vi "Begin.vi"(8 "error in":errorcluster) -> (0 "error out":errorcluster)   [LabVIEW 2016]
doc: "Called before other user functions, this VI is expected to open initial I/O refnums, load in file data, and do all program initialization. Notice that the <B>error out</B> terminal is simply used for data flow. Wiring it to other structures or subVIs ensures that this VI runs first."
uses:
  <vilib>/Rock Robotics/WPI/SafetyOutput/WPI_SafetyOutputConfigMenu.ctl
  <vilib>/Rock Robotics/WPI/DriverStation/WPI_DriverStationRobotMode2.ctl
  <vilib>/Rock Robotics/WPI/Joystick/WPI_JoystickDeviceEnum.ctl
  <vilib>/Rock Robotics/SystemInterfaces/DIO/FPGA_DIOPWMChannel.ctl
  <vilib>/Rock Robotics/SystemInterfaces/DIO/FPGA_DIOChannel.ctl
  <vilib>/Rock Robotics/SystemInterfaces/i2clib/i2c_bus.ctl
  <vilib>/Rock Robotics/SystemInterfaces/DIO/FPGA_DIORelayChannel.ctl
  <vilib>/Rock Robotics/WPI/Relay/WPI_RelayDirection.ctl
  <vilib>/Rock Robotics/WPI/Solenoid/WPI_SolenoidChannel.ctl
  <vilib>/Rock Robotics/WPI/ThirdParty/CanMotor/TalonSRX/WPI_CANTalonSRX_APIControlMode.ctl
  Robot Global Data.vi
  <vilib>/Rock Robotics/Network Tables/NT Write String Array.vi
  <vilib>/Rock Robotics/WPI/MotorControl/WPI_MotorControlOpen VictorSP.vi
  <vilib>/Rock Robotics/WPI/Switch/WPI_SwitchOpenLimit.vi
  <vilib>/Rock Robotics/WPI/RobotDrive/WPI_RobotDriveOpen4MotorWithVictorSP.vi
  <vilib>/Rock Robotics/WPI/Solenoid/WPI_SolenoidOpenSingle.vi
  <vilib>/Rock Robotics/WPI/Counter/WPI_CounterDigitalInputToDigitalSource.vi
  <vilib>/Rock Robotics/WPI/Counter/WPI_CounterOpen UpDown Mode.vi
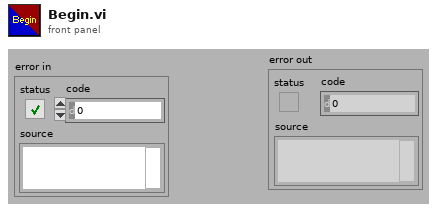
[diagram p1: front panel]
types:
  T1 = typedef "FPGA_DIOChannel.ctl" = enum8{"DIO 0", "DIO 1", "DIO 2", "DIO 3", "DIO 4", "DIO 5", "DIO 6", "DIO 7", "DIO 8", "DIO 9", "DIO MXP 0", "DIO MXP 1", "DIO MXP 2", "DIO MXP 3", "DIO MXP 4", "DIO MXP 5", "DIO MXP 6", "DIO MXP 7", "DIO MXP 8", "DIO MXP 9", "DIO MXP 10", "DIO MXP 11", "DIO MXP 12", "DIO MXP 13", "DIO MXP 14", "DIO MXP 15", "SPI Port CS1", "SPI Port CS2", "SPI Port CS3", "SPI Port MISO", "SPI Port MOSI", "Invalid"}
  T2 = typedef "WPI_SolenoidChannel.ctl" = enum8{"Solenoid 0", "Solenoid 1", "Solenoid 2", "Solenoid 3", "Solenoid 4", "Solenoid 5", "Solenoid 6", "Solenoid 7", "Invalid"}
  T3 = typedef "FPGA_DIOPWMChannel.ctl" = enum8{"PWM 0", "PWM 1", "PWM 2", "PWM 3", "PWM 4", "PWM 5", "PWM 6", "PWM 7", "PWM 8", "PWM 9", "PWM MXP 0", "PWM MXP 1", "PWM MXP 2", "PWM MXP 3", "PWM MXP 4", "PWM MXP 5", "PWM MXP 6", "PWM MXP 7", "PWM MXP 8", "PWM MXP 9", "Invalid"}
  T4 = typedef "WPI_CANTalonSRX_APIControlMode.ctl" = enum8{"Percent VBus", "Speed", "Position", "Slave", "Unchanged / Invalid", "Voltage Compensation", "Current", "Motion Profile", "Motion Magic"}
  T5 = typedef "FPGA_DIORelayChannel.ctl" = enum8{"Relay 0", "Relay 1", "Relay 2", "Relay 3", "Invalid"}
  T6 = typedef "WPI_RelayDirection.ctl" = enum16{"Both directions", "Forward only", "Reverse only"}
  T7 = typedef "i2c_bus.ctl" = enum16{"I2C On-Board", "I2C MXP", "Invalid"}
  T8 = typedef "WPI_JoystickDeviceEnum.ctl" = enum16{"USB 0", "USB 1", "USB 2", "USB 3", "USB 4", "USB 5"}
  T9 = typedef "WPI_DriverStationRobotMode2.ctl" = enum16{"Autonomous Disabled", "Autonomous Enabled", "Teleop Disabled", "Teleop Enabled", "Disconnected", "Finish", "Test Disabled", "Test Enabled", "Emergency Stopped"}
  T10 = typedef "WPI_SafetyOutputConfigMenu.ctl" = enum16{"Enable", "Disable"}
  T11 = typedef "WPI_JoystickDevRef.ctl" = cluster{"Device":T8}
  T12 = typedef "WPI_ServoDeviceRef.ctl" = cluster{"DeviceStatus":errorcluster, "PWM Channel":T3, "DeadBand":T13}
  T13 = typedef "WPI_PWMDeadband.ctl" = cluster{"Name":string, "maxPositivePwm":i32, "minPositivePwm":i32, "centerPwm":i32, "maxNegativePwm":i32, "minNegativePwm":i32, "angularRange":u16}
  T14 = typedef "WPI_MotorControlDeviceRef.ctl" = cluster{"DeviceStatus":errorcluster, "Type":T15, "PWM":cluster{"PWM Channel":T3, "DeadBand":T13}, "CAN":cluster{"Device Number":u8, "SetOutput VI Ref":variant, "GetOutput VI Ref":variant, "Enable VI Ref":variant, "Disable VI Ref":variant, "Data":variant}, "Invert":bool}
  T15 = typedef "WPI_MotorControlType.ctl" = enum16{"PWM", "CAN"}
  T16 = typedef "WPI_RobotDriveDevRef.ctl" = cluster{"DevStatus":errorcluster, "Motors[]":T14[], "Square Inputs":bool, "Max Output":dbl}
  T17 = typedef "WPI_SwitchDevRef.ctl" = cluster{"DevStatus":errorcluster, "DIO Channel":T1, "CntIndex":T18, "Normally Closed":bool}
  T18 = typedef "FPGA_CounterCtrSystemIndex.ctl" = enum8{"Ctr 0", "Ctr 1", "Ctr 2", "Ctr 3", "Ctr 4", "Ctr 5", "Ctr 6", "Ctr 7", "Invalid"}
  T19 = typedef "WPI_I2CDevRef.ctl" = cluster{"DevStatus":errorcluster, "Device Address":u8, "Handle":i32, "I2C Bus":T7}
  T20 = typedef "WPI_DigitalInputDevRef.ctl" = cluster{"DevStatus":errorcluster, "DIO Channel":T1}
  T21 = typedef "FPGA_CounterEncoderSourceConvertionLVSourceType.ctl" = cluster{"DevStatus":errorcluster, "AnalogTriggerMode?":bool, "DigitalMode":cluster{"DIO Channel":T22}, "AnalogTriggerMode":cluster{"AnalogTriggerIndex":T23, "OutputType":T24}}
  T22 = typedef "FPGA_DIODigitalSourceChannel.ctl" = enum8{"DIO 0", "DIO 1", "DIO 2", "DIO 3", "DIO 4", "DIO 5", "DIO 6", "DIO 7", "DIO 8", "DIO 9", "DIO MXP 0", "DIO MXP 1", "DIO MXP 2", "DIO MXP 3", "DIO MXP 4", "DIO MXP 5", "DIO MXP 6", "DIO MXP 7", "DIO MXP 8", "DIO MXP 9", "DIO MXP 10", "DIO MXP 11", "DIO MXP 12", "DIO MXP 13", "DIO MXP 14", "DIO MXP 15", "Disabled"}
  T23 = typedef "FPGA_AnalogTriggerIndex.ctl" = enum8{"Trig 0", "Trig 1", "Trig 2", "Trig 3", "Trig 4", "Trig 5", "Trig 6", "Trig 7", "Invalid"}
  T24 = typedef "FPGA_AnalogTriggerOutType.ctl" = enum16{"InWindow", "TriggerState", "Rising", "Falling"}
  T25 = typedef "WPI_CounterDevRef.ctl" = cluster{"DevStatus":errorcluster, "CntIndex":T18}
  T26 = typedef "WPI_RelayDevRef.ctl" = cluster{"DevStatus":errorcluster, "Relay Channel":T5, "Relay Direction":T6}
  T27 = typedef "WPI_SolenoidDevRef.ctl" = cluster{"DevStatus":errorcluster, "Pneumatics Control Module":u8, "Forward Solenoid Channel":T2, "Reverse Solenoid Channel":T2}
  T28 = typedef "WPI_EncoderDevRef.ctl" = cluster{"DevStatus":errorcluster, "EncoderIndex":T29, "CounterIndex":T18, "DistancePerCount":dbl, "Decoding Type":T30}
  T29 = typedef "FPGA_EncoderIdx.ctl" = enum8{"Enc 0", "Enc 1", "Enc 2", "Enc 3", "Enc 4", "Enc 5", "Enc 6", "Enc 7", "Invalid"}
  T30 = typedef "WPI_EncoderType.ctl" = enum16{"1x", "2x", "4x"}
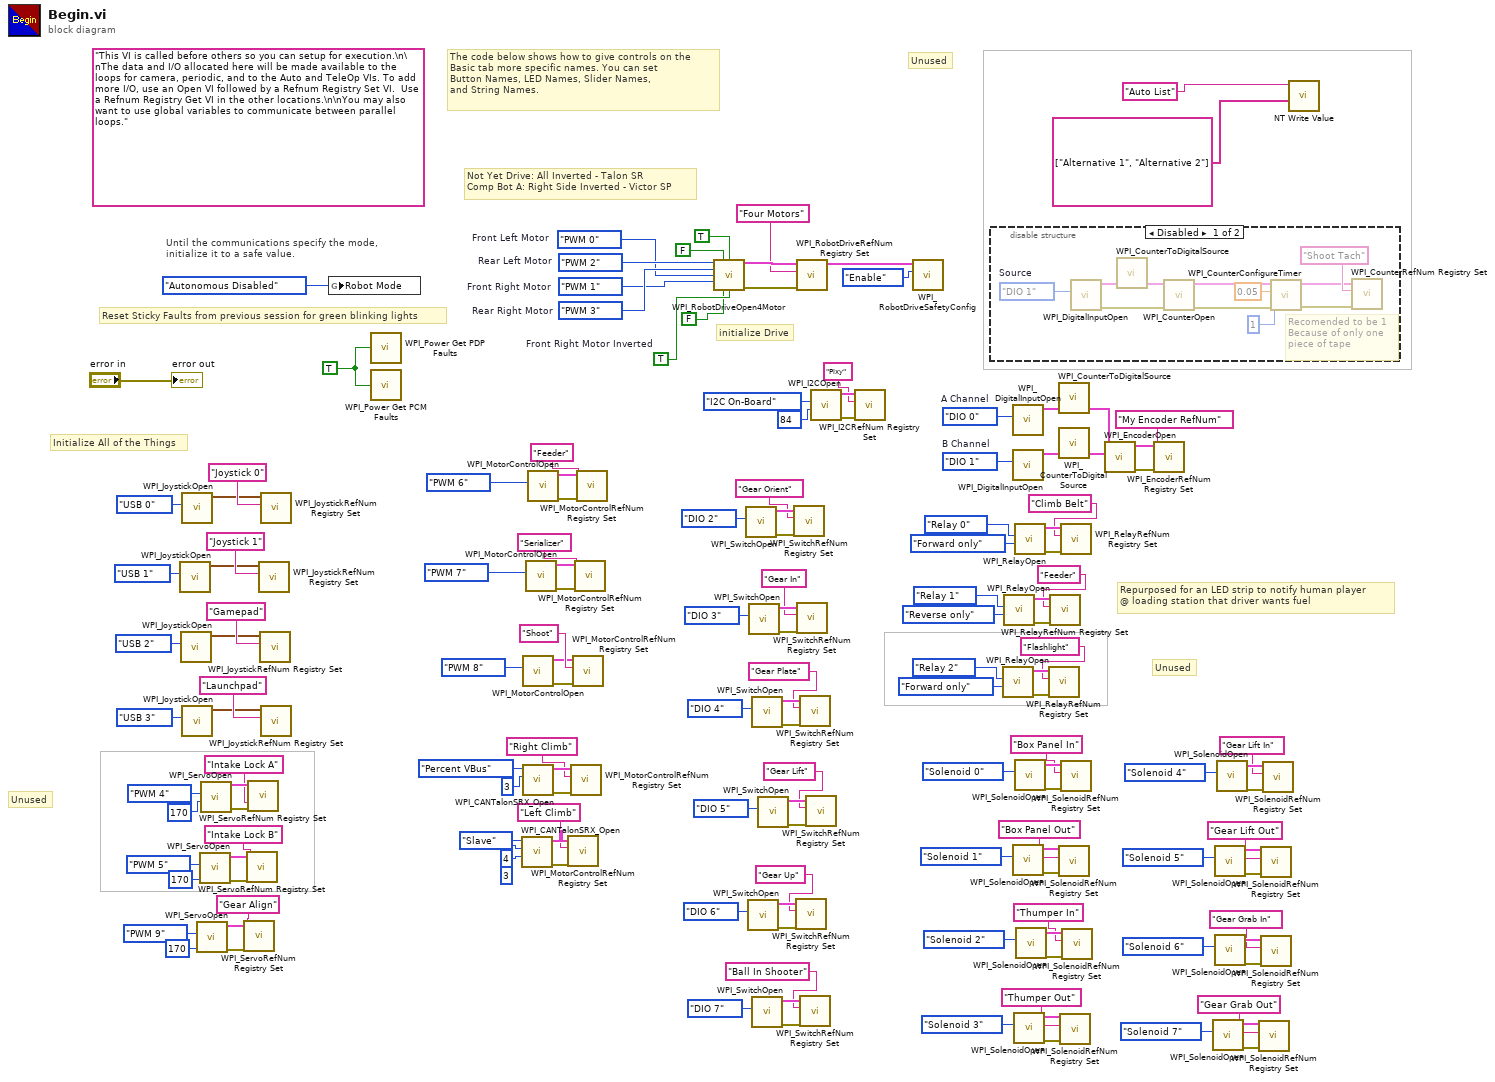
[diagram p0: block diagram]
diagram:
  w9 = FPGA_DIOChannel."DIO 1"  # B Channel
  w8 = FPGA_DIOChannel."DIO 0"  # A Channel
  w18 = TRUE
  w103 = TRUE  # Front Right Motor Inverted
  w141 = FPGA_DIOPWMChannel."PWM 1"  # Front Right Motor
  w142 = FPGA_DIOPWMChannel."PWM 0"  # Front Left Motor
  w143 = FPGA_DIOPWMChannel."PWM 3"  # Rear Right Motor
  w144 = FPGA_DIOPWMChannel."PWM 2"  # Rear Left Motor
  (unwired) "This VI is called before others so you can setup for execution.\n\nThe data and I/O allocated here will be made available to the loops for camera, periodic, and to the Auto and TeleOp VIs. To add more I/O, use an Open VI followed by a Refnum Registry Set VI.  Use a Refnum Registry Get VI in the other locations.\n\nYou may also want to use global variables to communicate between parallel loops."
  # "Repurposed for an LED strip to notify human player \n@ loading station that driver wants fuel"
  # "Reset Sticky Faults from previous session for green blinking lights"
  # "Unused"
  # "Unused"
  # "Unused"
  # "Not Yet Drive: All Inverted - Talon SR\nComp Bot A: Right Side Inverted - Victor SP"
  # "The code below shows how to give controls on the\nBasic tab more specific names. You can set\nButton Names, LED Names, Slider Names,\nand String Names."
  # "Initialize All of the Things"
  # "Until the communications specify the mode,\ninitialize it to a safe value."
  # "initialize Drive"
  n1 = call <vilib>:"WPI_JoystickOpen.vi"("JoystickDevice"=WPI_JoystickDeviceEnum."USB 1") -> ("JoystickDevRef"=w136:T11)  [unwired: 10 in]
  n2 = call <vilib>:"WPI_JoystickOpen.vi"("JoystickDevice"=WPI_JoystickDeviceEnum."USB 2") -> ("JoystickDevRef"=w133:T11)  [unwired: 10 in]
  n3 = call <vilib>:"WPI_JoystickOpen.vi"("JoystickDevice"=WPI_JoystickDeviceEnum."USB 0") -> ("JoystickDevRef"=w146:T11)  [unwired: 10 in]
  n4 = call <vilib>:"WPI_JoystickOpen.vi"("JoystickDevice"=WPI_JoystickDeviceEnum."USB 3") -> ("JoystickDevRef"=w130:T11)  [unwired: 10 in]
  n5 = call <vilib>:"WPI_ServoOpen.vi"("Angular Range"=u16 170, "PWM Channel"=FPGA_DIOPWMChannel."PWM 9") -> ("error out"=w66:errorcluster, "ServoDeviceRef"=w65:T12)  [unwired: 8 in]
  n6 = call <vilib>:"WPI_ServoOpen.vi"("Angular Range"=u16 170, "PWM Channel"=FPGA_DIOPWMChannel."PWM 5") -> ("error out"=w81:errorcluster, "ServoDeviceRef"=w80:T12)  [unwired: 8 in]
  n7 = call <vilib>:"WPI_ServoOpen.vi"("Angular Range"=u16 170, "PWM Channel"=FPGA_DIOPWMChannel."PWM 4") -> ("error out"=w84:errorcluster, "ServoDeviceRef"=w83:T12)  [unwired: 8 in]
  n8 = call <vilib>:"WPI_ServoRefNum Registry Set.vi"("error in (no error)"=w66, "refnum name"="Gear Align", "ServoDeviceRef"=w65) -> ()  [unwired: 7 in, 2 out]
  n9 = call <vilib>:"WPI_ServoRefNum Registry Set.vi"("error in (no error)"=w81, "refnum name"="Intake Lock B", "ServoDeviceRef"=w80) -> ()  [unwired: 7 in, 2 out]
  n10 = call <vilib>:"WPI_ServoRefNum Registry Set.vi"("error in (no error)"=w84, "refnum name"="Intake Lock A", "ServoDeviceRef"=w83) -> ()  [unwired: 7 in, 2 out]
  n11 = call <vilib>:"WPI_JoystickRefNum Registry Set.vi"("refnum name"="Joystick 1", "JoystickDevRef"=w136) -> ()  [unwired: 8 in, 2 out]
  n12 = call <vilib>:"WPI_JoystickRefNum Registry Set.vi"("refnum name"="Gamepad", "JoystickDevRef"=w133) -> ()  [unwired: 8 in, 2 out]
  n13 = call <vilib>:"WPI_JoystickRefNum Registry Set.vi"("refnum name"="Joystick 0", "JoystickDevRef"=w146) -> ()  [unwired: 8 in, 2 out]
  n14 = call <vilib>:"WPI_JoystickRefNum Registry Set.vi"("refnum name"="Launchpad", "JoystickDevRef"=w130) -> ()  [unwired: 8 in, 2 out]
  n15 = global write "Robot Global Data.vi" "Robot Mode"(WPI_DriverStationRobotMode2."Autonomous Disabled" ("Robot Mode")) -> ()
  n16 = call <vilib>:"WPI_Power Get PDP Faults.vi"("Clear Sticky Faults"=w18) -> ()  [unwired: 10 in, 5 out]
  n17 = call <vilib>:"WPI_Power Get PCM Faults.vi"("Clear Sticky Faults"=w18) -> ()  [unwired: 11 in, 4 out]
  n18 = call <vilib>:"WPI_CANTalonSRX_Open.vi"("Master Device Number"=u8 3, "Device Number"=u8 4, "Control Mode"=WPI_CANTalonSRX_APIControlMode."Slave") -> ("error out"=w59:errorcluster, "CAN Talon SRX Ref"=w58:T14)  [unwired: 7 in]
  n19 = call-poly <vilib>:"WPI_MotorControlOpen.vi"("PWM Channel"=FPGA_DIOPWMChannel."PWM 8") -> ("error out"=w49:errorcluster, "MotorControlDeviceRef"=w48:T14)  [unwired: 9 in]
  n20 = call <vilib>:"WPI_CANTalonSRX_Open.vi"("Device Number"=u8 3, "Control Mode"=WPI_CANTalonSRX_APIControlMode."Percent VBus") -> ("error out"=w61:errorcluster, "CAN Talon SRX Ref"=w60:T14)  [unwired: 8 in]
  n21 = call-poly <vilib>:"WPI_MotorControlOpen.vi"("PWM Channel"=FPGA_DIOPWMChannel."PWM 7") -> ("error out"=w124:errorcluster, "MotorControlDeviceRef"=w123:T14)  [unwired: 9 in]
  n22 = call-poly <vilib>:"WPI_MotorControlOpen.vi"("PWM Channel"=FPGA_DIOPWMChannel."PWM 6") -> ("error out"=w128:errorcluster, "MotorControlDeviceRef"=w127:T14)  [unwired: 9 in]
  n23 = call <vilib>:"WPI_MotorControlRefNum Registry Set.vi"("error in (no error)"=w59, "refnum name"="Left Climb", "MotorControlDevRef"=w58) -> ()  [unwired: 7 in, 2 out]
  n24 = call <vilib>:"WPI_MotorControlRefNum Registry Set.vi"("error in (no error)"=w61, "refnum name"="Right Climb", "MotorControlDevRef"=w60) -> ()  [unwired: 7 in, 2 out]
  n25 = call <vilib>:"WPI_MotorControlRefNum Registry Set.vi"("error in (no error)"=w49, "refnum name"="Shoot", "MotorControlDevRef"=w48) -> ()  [unwired: 7 in, 2 out]
  n26 = call <vilib>:"WPI_MotorControlRefNum Registry Set.vi"("error in (no error)"=w124, "refnum name"="Serializer", "MotorControlDevRef"=w123) -> ()  [unwired: 7 in, 2 out]
  n27 = call <vilib>:"WPI_MotorControlRefNum Registry Set.vi"("error in (no error)"=w128, "refnum name"="Feeder", "MotorControlDevRef"=w127) -> ()  [unwired: 7 in, 2 out]
  n28 = call-poly <vilib>:"WPI_RobotDriveOpen4Motor.vi"("Rear Left Motor"=w144, "Rear Left Motor Inverted"=FALSE, "Rear Right Motor Inverted"=TRUE, "Rear Right Motor"=w143, "Front Left Motor"=w142, "Front Right Motor"=w141, "Front Left Motor Inverted"=FALSE, "Front Right Motor Inverted"=w103) -> ("RobotDriveDevRef"=w153:T16, "error out"=w151:errorcluster)  [unwired: 6 in]
  n29 = call-poly <vilib>:"WPI_SwitchOpen.vi"("DIO Channel"=FPGA_DIOChannel."DIO 2") -> ("error out"=w120:errorcluster, "SwitchDevRef"=w119:T17)  [unwired: 9 in]
  n30 = call-poly <vilib>:"WPI_SwitchOpen.vi"("DIO Channel"=FPGA_DIOChannel."DIO 6") -> ("error out"=w17:errorcluster, "SwitchDevRef"=w16:T17)  [unwired: 9 in]
  n31 = call-poly <vilib>:"WPI_SwitchOpen.vi"("DIO Channel"=FPGA_DIOChannel."DIO 3") -> ("error out"=w116:errorcluster, "SwitchDevRef"=w115:T17)  [unwired: 9 in]
  n32 = call-poly <vilib>:"WPI_SwitchOpen.vi"("DIO Channel"=FPGA_DIOChannel."DIO 4") -> ("error out"=w112:errorcluster, "SwitchDevRef"=w111:T17)  [unwired: 9 in]
  n33 = call-poly <vilib>:"WPI_SwitchOpen.vi"("DIO Channel"=FPGA_DIOChannel."DIO 7") -> ("error out"=w13:errorcluster, "SwitchDevRef"=w12:T17)  [unwired: 9 in]
  n34 = call-poly <vilib>:"WPI_SwitchOpen.vi"("DIO Channel"=FPGA_DIOChannel."DIO 5") -> ("error out"=w22:errorcluster, "SwitchDevRef"=w21:T17)  [unwired: 9 in]
  n35 = call <vilib>:"WPI_SwitchRefNum Registry Set.vi"("error in (no error)"=w120, "refnum name"="Gear Orient", "SwitchDevRef"=w119) -> ()  [unwired: 7 in, 2 out]
  n36 = call <vilib>:"WPI_SwitchRefNum Registry Set.vi"("error in (no error)"=w17, "refnum name"="Gear Up", "SwitchDevRef"=w16) -> ()  [unwired: 7 in, 2 out]
  n37 = call <vilib>:"WPI_RobotDriveRefNum Registry Set.vi"("error in (no error)"=w151, "refnum name"="Four Motors", "RobotDriveDevRef"=w153) -> ("RobotDriveDevRef"=w150:T16)  [unwired: 1 in, 7 out]
  n38 = call <vilib>:"WPI_SwitchRefNum Registry Set.vi"("error in (no error)"=w116, "refnum name"="Gear In", "SwitchDevRef"=w115) -> ()  [unwired: 7 in, 2 out]
  n39 = call <vilib>:"WPI_SwitchRefNum Registry Set.vi"("error in (no error)"=w112, "refnum name"="Gear Plate", "SwitchDevRef"=w111) -> ()  [unwired: 7 in, 2 out]
  n40 = call <vilib>:"WPI_SwitchRefNum Registry Set.vi"("error in (no error)"=w13, "refnum name"="Ball In Shooter", "SwitchDevRef"=w12) -> ()  [unwired: 7 in, 2 out]
  n41 = call <vilib>:"WPI_SwitchRefNum Registry Set.vi"("error in (no error)"=w22, "refnum name"="Gear Lift", "SwitchDevRef"=w21) -> ()  [unwired: 7 in, 2 out]
  n42 = call <vilib>:"WPI_I2COpen.vi"("Device Address"=u8 84, "I2C Bus"=i2c_bus."I2C On-Board") -> ("error out"=w108:errorcluster, "I2CDevRef"=w107:T19)  [unwired: 8 in]
  n43 = call <vilib>:"WPI_I2CRefNum Registry Set.vi"("error in (no error)"=w108, "refnum name"="Pixy", "I2CDevRef"=w107) -> ()  [unwired: 7 in, 2 out]
  n44 = call <vilib>:"WPI_RobotDriveSafetyConfig.vi"("mode"=WPI_SafetyOutputConfigMenu."Enable", "RobotDriveDevRef"=w150) -> ()  [unwired: 8 in, 2 out]
  n45 = disable-structure shown="Disabled" {
    frame Disabled {
      w163 = FPGA_DIOChannel."DIO 1"  # Source
      # "Recomended to be 1\nBecause of only one \npiece of tape"
      n46 = call <vilib>:"WPI_DigitalInputOpen.vi"("DIO Channel"=w163) -> ("error out"=w158:errorcluster, "DigitalInputDevRef"=w162:T20)  [unwired: 1 in, 8 out]
      n47 = call-poly <vilib>:"WPI_CounterToDigitalSource.vi"("DigitalInputDevRef"=w162) -> ("Digital Source"=w164:T21)  [unwired: 6 out]
      n48 = call-poly <vilib>:"WPI_CounterOpen.vi"("error in (no error)"=w158, "Up Source"=w164) -> ("error out"=w160:errorcluster, "CounterDevRef"=w159:T25)  [unwired: 5 in, 3 out]
      n49 = call <vilib>:"WPI_CounterConfigureTimer.vi"("error in (no error)"=w160, "Number Samples to Average"=u8 1, "MaxPeriod (sec)"=0.05, "CounterDevRef in"=w159) -> ("error out"=w154:errorcluster, "CounterDevRef out"=w155:T25)  [unwired: 6 in]
      n50 = call <vilib>:"WPI_CounterRefNum Registry Set.vi"("error in (no error)"=w154, "refnum name"="Shoot Tach", "CounterDevRef"=w155) -> ()  [unwired: 7 in, 2 out]
    }
    frame Enabled {
    }
  }
  n51 = call <vilib>:"WPI_RelayOpen.vi"("Relay Direction"=WPI_RelayDirection."Forward only", "Relay Channel"=FPGA_DIORelayChannel."Relay 2") -> ("error out"=w99:errorcluster, "RelayDevRef"=w98:T26)  [unwired: 8 in]
  n52 = call <vilib>:"WPI_RelayOpen.vi"("Relay Direction"=WPI_RelayDirection."Reverse only", "Relay Channel"=FPGA_DIORelayChannel."Relay 1") -> ("error out"=w89:errorcluster, "RelayDevRef"=w88:T26)  [unwired: 8 in]
  n53 = call <vilib>:"WPI_DigitalInputOpen.vi"("DIO Channel"=w8) -> ("DigitalInputDevRef"=w5:T20)  [unwired: 1 in, 9 out]
  n54 = call <vilib>:"WPI_DigitalInputOpen.vi"("DIO Channel"=w9) -> ("DigitalInputDevRef"=w6:T20)  [unwired: 1 in, 9 out]
  n55 = call-poly <vilib>:"WPI_SolenoidOpen.vi"("Solenoid Channel"=WPI_SolenoidChannel."Solenoid 1") -> ("error out"=w70:errorcluster, "SolenoidDevRef"=w69:T27)  [unwired: 9 in]
  n56 = call-poly <vilib>:"WPI_SolenoidOpen.vi"("Solenoid Channel"=WPI_SolenoidChannel."Solenoid 3") -> ("error out"=w42:errorcluster, "SolenoidDevRef"=w41:T27)  [unwired: 9 in]
  n57 = call <vilib>:"WPI_RelayOpen.vi"("Relay Direction"=WPI_RelayDirection."Forward only", "Relay Channel"=FPGA_DIORelayChannel."Relay 0") -> ("error out"=w94:errorcluster, "RelayDevRef"=w93:T26)  [unwired: 8 in]
  n58 = call-poly <vilib>:"WPI_SolenoidOpen.vi"("Solenoid Channel"=WPI_SolenoidChannel."Solenoid 0") -> ("error out"=w74:errorcluster, "SolenoidDevRef"=w73:T27)  [unwired: 9 in]
  n59 = call-poly <vilib>:"WPI_SolenoidOpen.vi"("Solenoid Channel"=WPI_SolenoidChannel."Solenoid 2") -> ("error out"=w46:errorcluster, "SolenoidDevRef"=w45:T27)  [unwired: 9 in]
  n60 = call <vilib>:"WPI_RelayRefNum Registry Set.vi"("error in (no error)"=w99, "refnum name"="Flashlight", "RelayDevRef"=w98) -> ()  [unwired: 7 in, 2 out]
  n61 = call <vilib>:"WPI_RelayRefNum Registry Set.vi"("error in (no error)"=w89, "refnum name"="Feeder", "RelayDevRef"=w88) -> ()  [unwired: 7 in, 2 out]
  n62 = call-poly <vilib>:"WPI_CounterToDigitalSource.vi"("DigitalInputDevRef"=w5) -> ("Digital Source"=w4:T21)  [unwired: 6 out]
  n63 = call-poly <vilib>:"WPI_CounterToDigitalSource.vi"("DigitalInputDevRef"=w6) -> ("Digital Source"=w7:T21)  [unwired: 6 out]
  n64 = call <vilib>:"WPI_SolenoidRefNum Registry Set.vi"("error in (no error)"=w70, "refnum name"="Box Panel Out", "SolenoidDevRef"=w69) -> ()  [unwired: 7 in, 2 out]
  n65 = call <vilib>:"WPI_SolenoidRefNum Registry Set.vi"("error in (no error)"=w42, "refnum name"="Thumper Out", "SolenoidDevRef"=w41) -> ()  [unwired: 7 in, 2 out]
  n66 = call <vilib>:"WPI_RelayRefNum Registry Set.vi"("error in (no error)"=w94, "refnum name"="Climb Belt", "RelayDevRef"=w93) -> ()  [unwired: 7 in, 2 out]
  n67 = call <vilib>:"WPI_SolenoidRefNum Registry Set.vi"("error in (no error)"=w74, "refnum name"="Box Panel In", "SolenoidDevRef"=w73) -> ()  [unwired: 7 in, 2 out]
  n68 = call <vilib>:"WPI_SolenoidRefNum Registry Set.vi"("error in (no error)"=w46, "refnum name"="Thumper In", "SolenoidDevRef"=w45) -> ()  [unwired: 7 in, 2 out]
  n69 = call <vilib>:"WPI_EncoderOpen.vi"("BSource"=w7, "ASource"=w4) -> ("error out"=w3:errorcluster, "EncoderDevRef"=w2:T28)  [unwired: 6 in, 2 out]
  n70 = call <vilib>:"WPI_EncoderRefNum Registry Set.vi"("error in (no error)"=w3, "refnum name"="My Encoder RefNum", "EncoderDevRef"=w2) -> ()  [unwired: 7 in, 2 out]
  n71 = call-poly <vilib>:"WPI_SolenoidOpen.vi"("Solenoid Channel"=WPI_SolenoidChannel."Solenoid 7") -> ("error out"=w26:errorcluster, "SolenoidDevRef"=w25:T27)  [unwired: 9 in]
  n72 = call-poly <vilib>:"WPI_SolenoidOpen.vi"("Solenoid Channel"=WPI_SolenoidChannel."Solenoid 5") -> ("error out"=w34:errorcluster, "SolenoidDevRef"=w33:T27)  [unwired: 9 in]
  n73 = call-poly <vilib>:"WPI_SolenoidOpen.vi"("Solenoid Channel"=WPI_SolenoidChannel."Solenoid 6") -> ("error out"=w30:errorcluster, "SolenoidDevRef"=w29:T27)  [unwired: 9 in]
  n74 = call-poly <vilib>:"WPI_SolenoidOpen.vi"("Solenoid Channel"=WPI_SolenoidChannel."Solenoid 4") -> ("error out"=w38:errorcluster, "SolenoidDevRef"=w37:T27)  [unwired: 9 in]
  n75 = call <vilib>:"WPI_SolenoidRefNum Registry Set.vi"("error in (no error)"=w26, "refnum name"="Gear Grab Out", "SolenoidDevRef"=w25) -> ()  [unwired: 7 in, 2 out]
  n76 = call <vilib>:"WPI_SolenoidRefNum Registry Set.vi"("error in (no error)"=w34, "refnum name"="Gear Lift Out", "SolenoidDevRef"=w33) -> ()  [unwired: 7 in, 2 out]
  n77 = call <vilib>:"WPI_SolenoidRefNum Registry Set.vi"("error in (no error)"=w30, "refnum name"="Gear Grab In", "SolenoidDevRef"=w29) -> ()  [unwired: 7 in, 2 out]
  n78 = call <vilib>:"WPI_SolenoidRefNum Registry Set.vi"("error in (no error)"=w38, "refnum name"="Gear Lift In", "SolenoidDevRef"=w37) -> ()  [unwired: 7 in, 2 out]
  n79 = call-poly <vilib>:"NT Write Value.vi"("String Array"=string[] ["Alternative 1", "Alternative 2"], "Name"="Auto List") -> ()  [unwired: 9 in, 1 out]
  "error out" <- "error in"
